vi "Load Provider.vi"(8 "error in":errorcluster, 10 "Name":string, 11 "Configuration UI Actor in":refnum<class "Configuration UI Actor.lvclass">) -> (0 "error out":errorcluster, 3 "Configuration UI Actor out":refnum<class "Configuration UI Actor.lvclass">)   [LabVIEW 2023, in "Configuration UI Actor.lvlib" / "Configuration UI Actor.lvclass"]
uses:
  Configuration UI Actor.lvclass
  <vilib>/MGI/Panel Manager/Panel Actor/Panel Actor/Panel Actor.lvclass
  Configuration UI Actor.lvclass/Configuration UI Actor.ctl
  <vilib>/ActorFramework/Message Enqueuer/Message Enqueuer.lvclass/Message Enqueuer.ctl
  <vilib>/ActorFramework/Message Enqueuer/Enqueue.vi
  <vilib>/MGI/Panel Manager/Panel/Panel/Subpanel/Subpanel.lvclass
  <vilib>/ActorFramework/Stop Msg/Stop Msg.lvclass
  <vilib>/Utility/LVClass/Get LV Class Name.vi
  <resource>/AFDebug/Generate Trace for Message.vi
  <vilib>/ActorFramework/Message Priority Queue/Priority Enqueue.vi
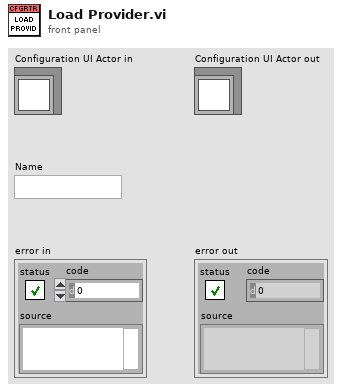
[diagram p1: front panel]
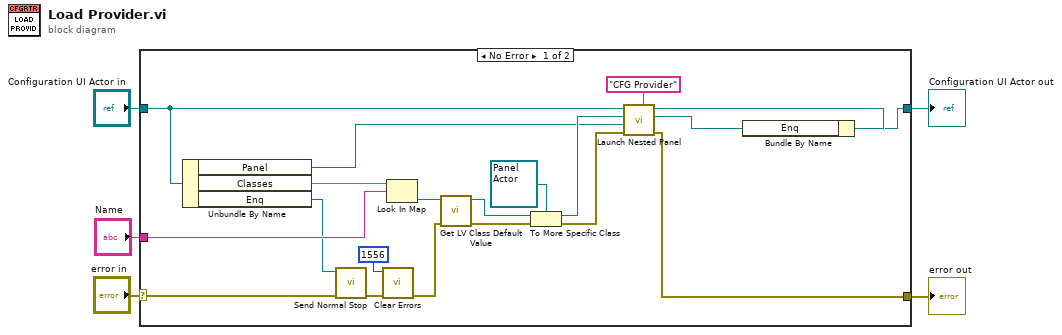
[diagram p0: block diagram]
diagram:
  n1 = case shown="No Error" "error in" {
    selector: "error in" -> [w10 w27]
    tunnel: [w16 w27] -> w4
    tunnel: [w13 w26] -> w2
    tunnel: "Configuration UI Actor in" -> [w18 w26]
    tunnel: "Name" -> [w24 _]
    frame No Error {
      n2 = Unbundle By Name(w18) -> ("Panel"=w15:refnum<class "Subpanel.lvclass">, "Classes"=w25:map{string, path}, "Enq"=w8:refnum<class "Message Enqueuer.lvclass">)
      n3 = call <vilib>:"Send Normal Stop.vi"("error in (no error)"=w10, "Message Enqueuer"=w8) -> ("error out"=w9:errorcluster)  [unwired: 9 in]
      n4 = call <vilib>:"Clear Errors.vi"("error in (no error)"=w9, "specific error code to clear (0: all)"=1556) -> ("error out"=w7:errorcluster)  [unwired: 4 in, 1 out]
      n5 = Look In Map(map=w25, key=w24) -> (value=w23:path)  [unwired: 1 in, 1 out]
      n6 = call <vilib>:"Get LV Class Default Value.vi"("error in (no error)"=w7, "class path"=w23) -> ("error out"=w21:errorcluster, "object"=w22:refnum<class>)  [unwired: 8 in]
      n7 = To More Specific Class(target class=refnum<class "Panel Actor.lvclass"> refnum ("Panel Actor in"), reference=w22, error in=w21) -> (specific class reference=w20:refnum<class "Panel Actor.lvclass">, error out=w17:errorcluster)
      n8 = call <vilib>:"Launch Nested Panel.vi"("Debug Alias"="CFG Provider", "error in (no error)"=w17, "Panel"=w15, "Nested Panel Actor"=w20, "Panel Actor in"=w18) -> ("error out"=w16:errorcluster, "Nested Actor's Enqueuer"=w12:refnum<class "Message Enqueuer.lvclass">, "Panel Actor out"=w14:refnum<class "Configuration UI Actor.lvclass">)  [unwired: 3 in, 1 out]
      n9 = Bundle By Name(cluster=w14, "Enq"=w12) -> (w13:refnum<class "Configuration UI Actor.lvclass">)
    }
    frame Error {
    }
  }
  "error out" <- w4
  "Configuration UI Actor out" <- w2
